vi "API - Add Tx Channel.vi"(6 "Data Type":T1, 8 "error in (no error)":errorcluster, 9 "Destination Ref":T2=18446744073709551615 format="%.0x", 10 "Channel Name":string, 11 "Item Ref In":T2=18446744073709551615 format="%.0x") -> (0 "error out":errorcluster, 2 "New Channel Ref":T2=18446744073709551615 format="%.0x", 3 "Item Ref Out":T2=18446744073709551615 format="%.0x")   [LabVIEW 2015]
uses:
  <vilib>/NI Veristand/Custom Device API/Custom Device Item Ref.ctl
  Shared/DataTypes.ctl
  <vilib>/NI Veristand/Custom Device API/Custom Device Channel.ctl
  <vilib>/NI Veristand/Custom Device API/Custom Device Channel Type.ctl
  Shared/Constants.vi
  <vilib>/NI VeriStand/Custom Device API/Custom Device API.lvlib
  Shared/UDP-Custom-Device Shared.lvlib
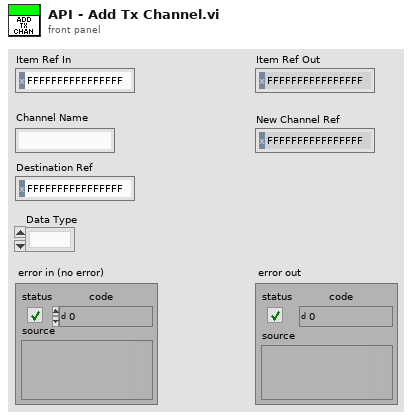
[diagram p1: front panel]
types:
  T1 = typedef "UDP-Custom-Device Shared.lvlib/DataTypes.ctl" = enum16{""}
  T2 = typedef "Custom Device API.lvlib/Custom Device Item Ref.ctl" = u64
  T3 = typedef "Custom Device API.lvlib/Custom Device Channel.ctl" = cluster{"Type":T4, "Units":string, "Default Value":dbl, "Faultable":bool, "Scalable":bool}
  T4 = typedef "Custom Device API.lvlib/Custom Device Channel Type.ctl" = enum16{"Input", "Output"}
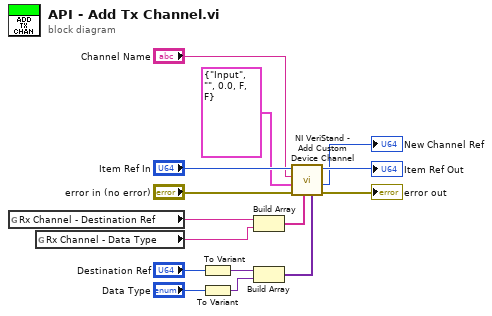
[diagram p0: block diagram]
diagram:
  n1 = global read "Constants.vi" "Rx Channel - Destination Ref"() -> (w3:string)
  n2 = global read "Constants.vi" "Rx Channel - Data Type"() -> (w2:string)
  n3 = To Variant(anything="Destination Ref") -> (Variant=w6:variant)
  n4 = To Variant(anything="Data Type") -> (Variant=w5:variant)
  n5 = Build Array(w3, w2) -> (w1:string[])
  n6 = Build Array(w6, w5) -> (w4:variant[])
  n7 = call <vilib>:"NI VeriStand - Add Custom Device Channel.vi"("Property Values"=w4, "Property names"=w1, "error in (no error)"="error in (no error)", "Channel"=T3 {"Type"=enum."Input", "Units"="", "Default Value"=0.0, "Faultable"=FALSE, "Scalable"=FALSE}, "Channel Name"="Channel Name", "Parent Ref in"="Item Ref In") -> ("error out"=→"error out":errorcluster, "Channel Ref"=→"New Channel Ref":T2, "Parent Ref out"=→"Item Ref Out":T2)  [unwired: 2 in, 1 out]
